vi "TEST Calibrate.vi"() -> ()   [LabVIEW 2010]
panel:
  in  "X In":dbl
  out "lo(x)":u16
  out "hi(x)":u16
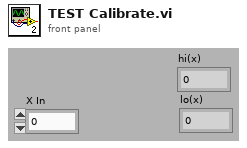
[diagram p1: front panel]
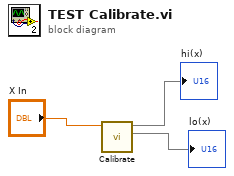
[diagram p0: block diagram]
diagram:
  n1 = call "Calibrate.vi"("X In"="X In") -> (9:→"lo(x)", 10:→"hi(x)")  [unwired: 7 in, 1 out]
